vi "GUI_kHz_AlpaoWFS_broken.vi"() -> ()   [LabVIEW 2020]
uses:
  Shared/GUI_Template/GUI_master/tcp new data cluster.ctl
  <vilib>/vision/NI_Vision_Development_Module.lvlib
  <vilib>/vision/Image Controls.llb/IMAQ Image.ctl
  Shared/GUI_Template/GUI_master/tcp_new_data_event.ctl
panel:
  out "SpatialImage::1":T1(plugin-control) caption="Spatial Image"
  out "retrievedFrogTrace::1":T1(plugin-control) caption="Retrieved Frog Trace"
  out "frogTrace::1":T1(plugin-control) caption="FROG Trace"
  in  "cameraselect::1":enum16{"temporal CAM", "spatial CAM"}(ring) caption="Select Camera"
  in  "exposure::1":dbl=0.001 caption="Exposure" min=0.001 max=10000.0 format="%_4p"
  in  "triggermode::1":bool caption="Blank Button"
  in  "Select device":string(combo)="kHz_WFS_Alpao"
  out "tcp data event 2":T2
  out "Tank":dbl(slide) scale=0.0..255.0 scale format="%#_6p"
  out "Rotated_spatial":T1(plugin-control) caption="Raw image"
  out "error out":errorcluster
  in  "UDP error message":string
  in  "Refresh Button":bool
  out "GUIdevice 1":string="kHz_WFS_Alpao"
  in  "insert tag":bool=TRUE
  in  "stop":bool
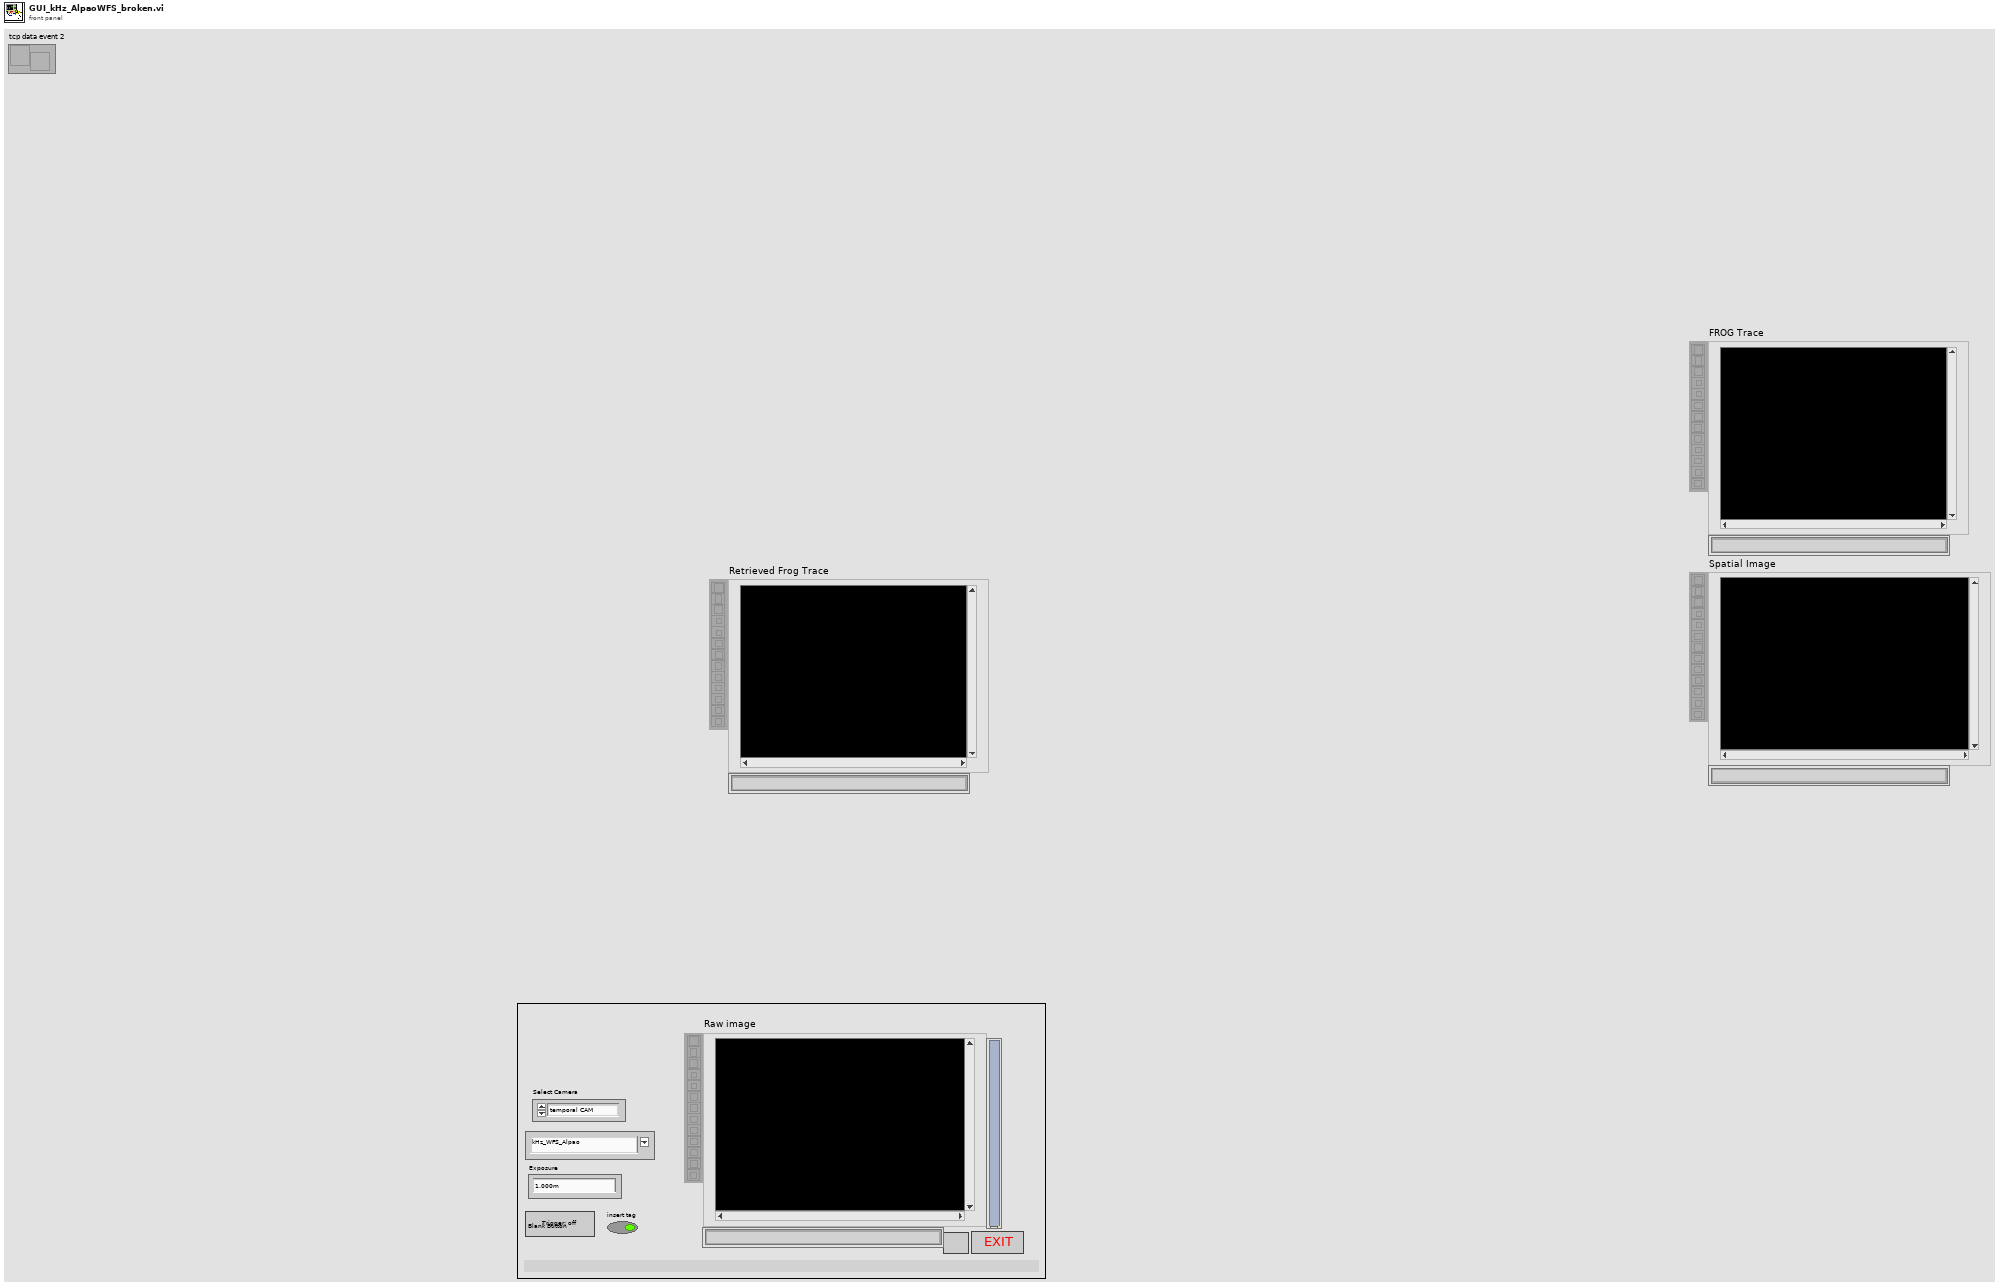
[diagram p1: front panel]
types:
  T1 = typedef "IMAQ Image.ctl" = refnum<image>
  T2 = typedef "tcp_new_data_event.ctl" = refnum<user-event>
  T3 = enum32{"invalid app kind", "Development System", "Run Time System", "Student Edition", "Embedded LabVIEW", "Evaluation", "Custom"}
  T4 = typedef "tcp new data cluster.ctl" = cluster{"EventEnum":enum16{"new data", "connection status update"}, "Device name":string}
  T5 = enum32{"Invalid", "Standard", "Closed", "Hidden", "Minimized", "Maximized"}
  T6 = cluster{"Left":i32, "Top":i32, "Right":i32, "Bottom":i32}
  T7 = cluster{"Core":cluster{"Current VI Reference":refnum<vi>, "Close Panel on Exit?":bool}, "Your Boolean data":bool, "Your string data":string, "SuperGUI":cluster{"STOP queue":refnum<queue>, "SuperGUI ref":refnum<vi>, "event reg":refnum<event-registration>}, "Images":cluster{"frogTrace::1":T1, "retrievedFrogTrace::1":T1, "SpatialImage::1":T1, "rotated_Temporal":T1, "rotated_Spatial":T1}}
  T8 = cluster{"frogTrace::1":T1, "retrievedFrogTrace::1":T1, "SpatialImage::1":T1, "rotated_Temporal":T1, "rotated_Spatial":T1}
  T9 = cluster{"STOP queue":refnum<queue>, "SuperGUI ref":refnum<vi>, "event reg":refnum<event-registration>}
  T10 = cluster{"Current VI Reference":refnum<vi>, "Close Panel on Exit?":bool}
  T11 = typedef "Image Type" = u32
  T12 = cluster{"histogram":u32[], "Minimal Value":sgl, "Maximal Value":sgl, "Starting Value":sgl, "Interval Width":sgl, "Mean Value":sgl, "Standard  Variation":sgl, "Area (pixels)":i32}
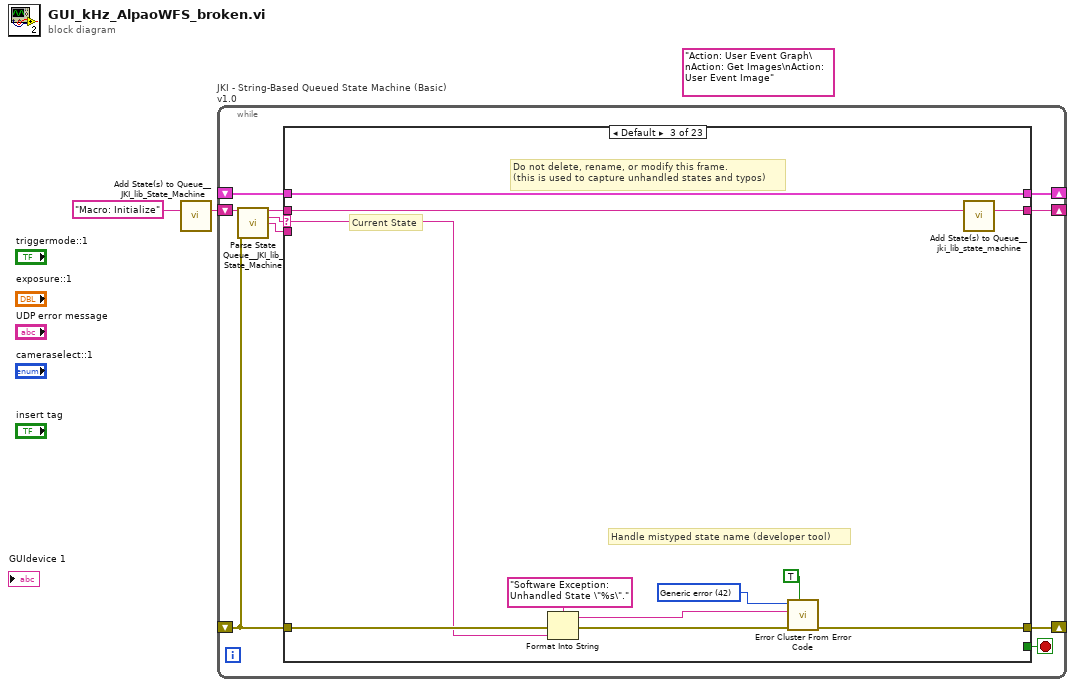
[diagram p0: block diagram]
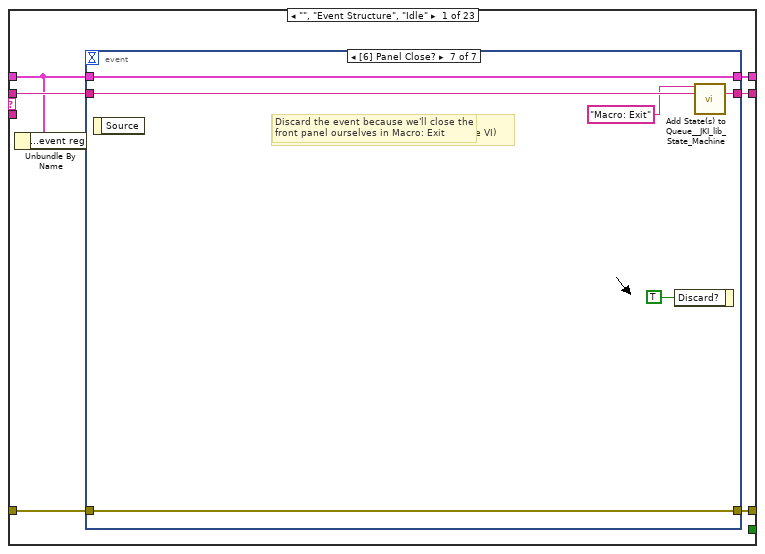
[diagram p2: hidden frame]
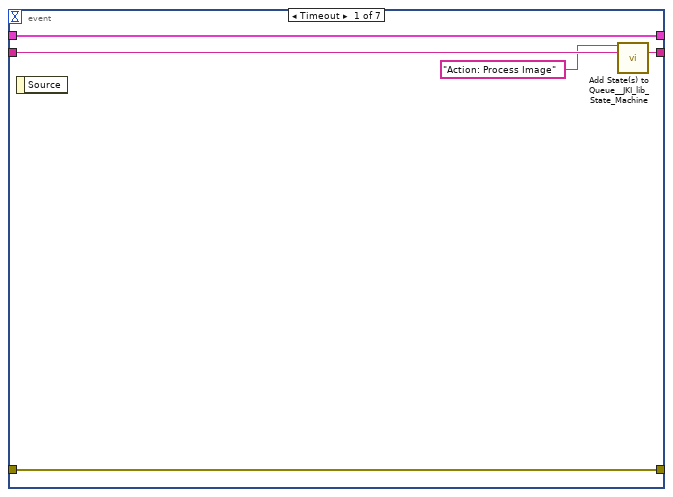
[diagram p3: hidden frame]
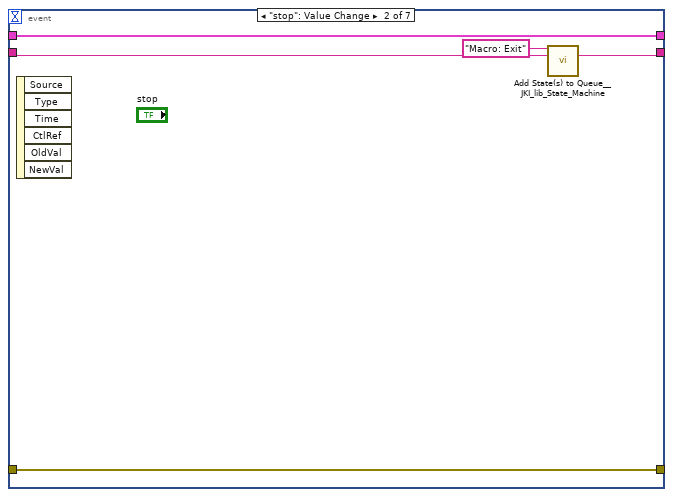
[diagram p4: hidden frame]
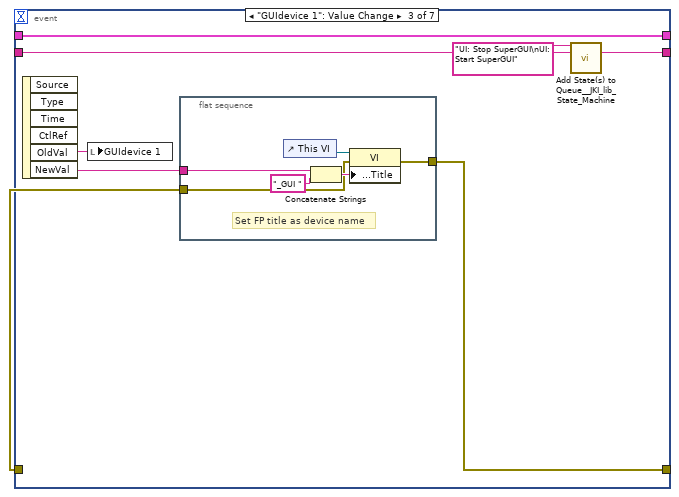
[diagram p5: hidden frame]
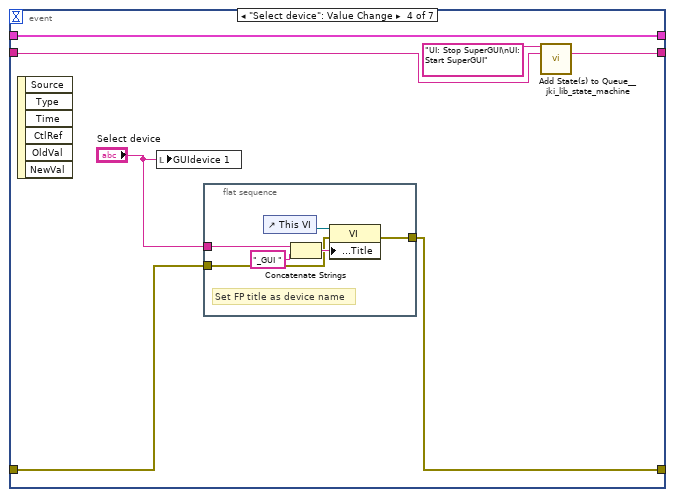
[diagram p6: hidden frame]
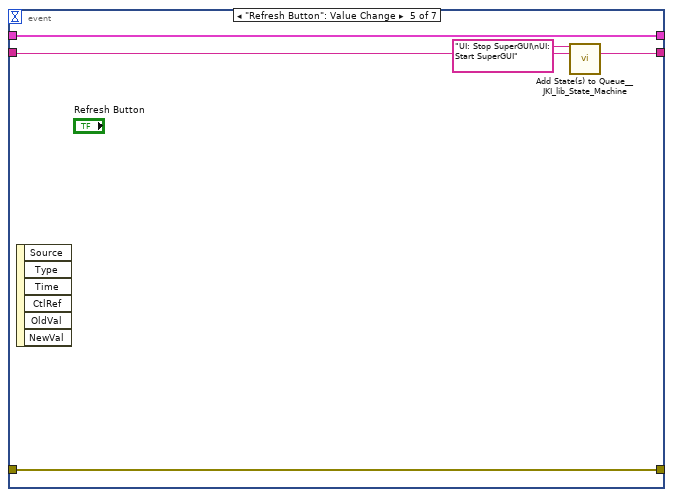
[diagram p7: hidden frame]
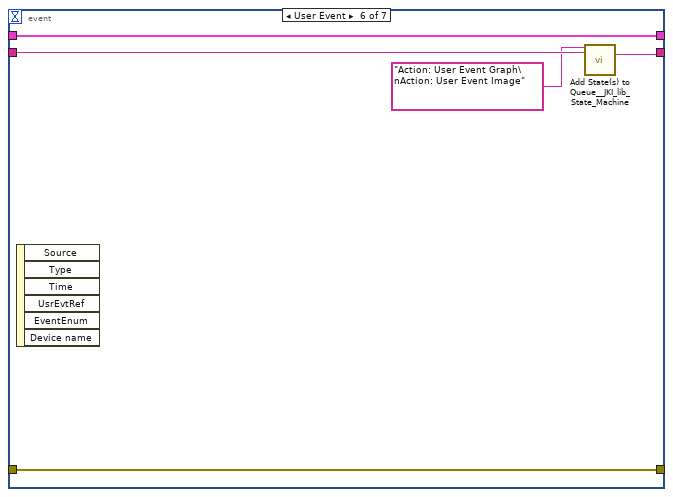
[diagram p8: hidden frame]
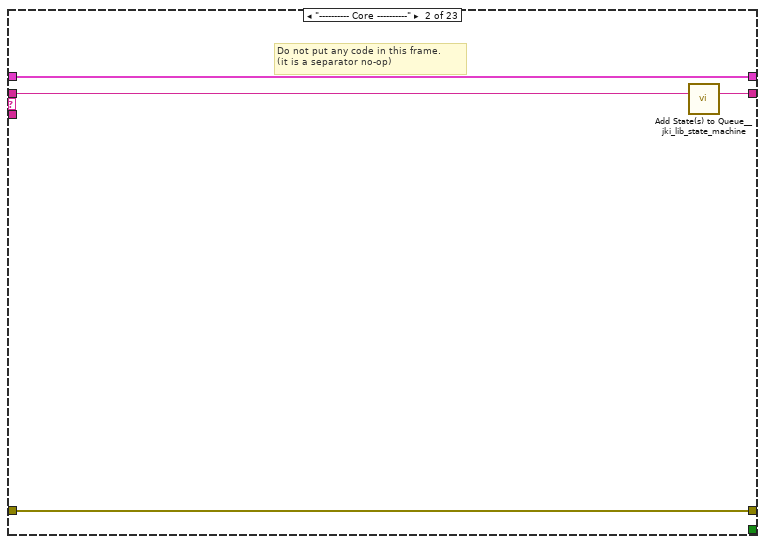
[diagram p9: hidden frame]
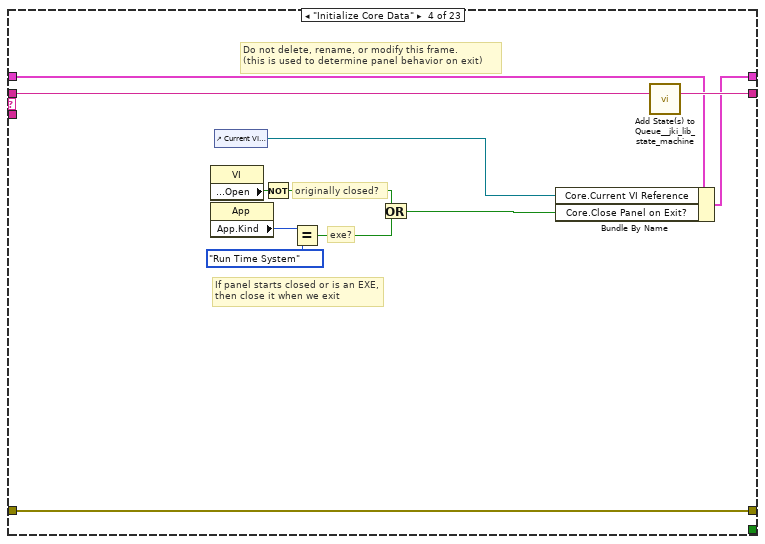
[diagram p10: hidden frame]
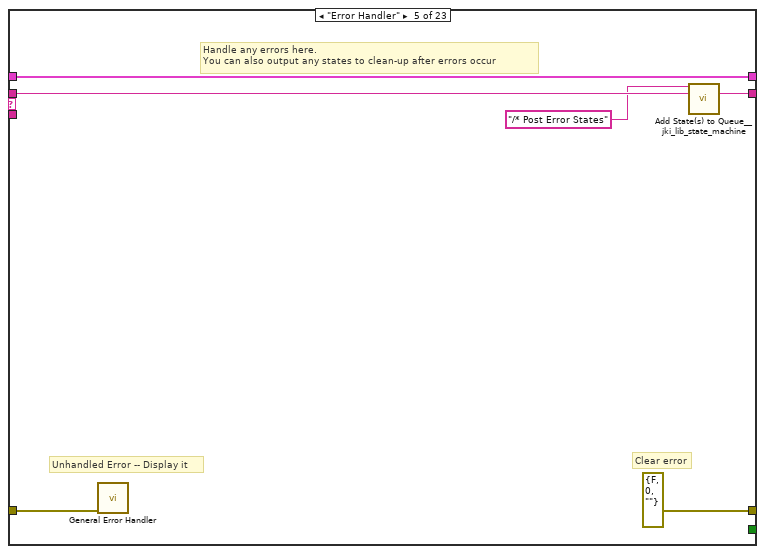
[diagram p11: hidden frame]
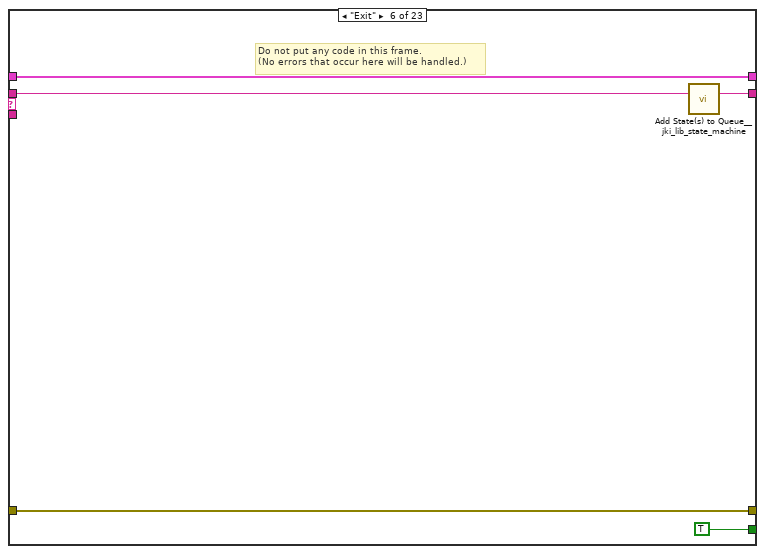
[diagram p12: hidden frame]
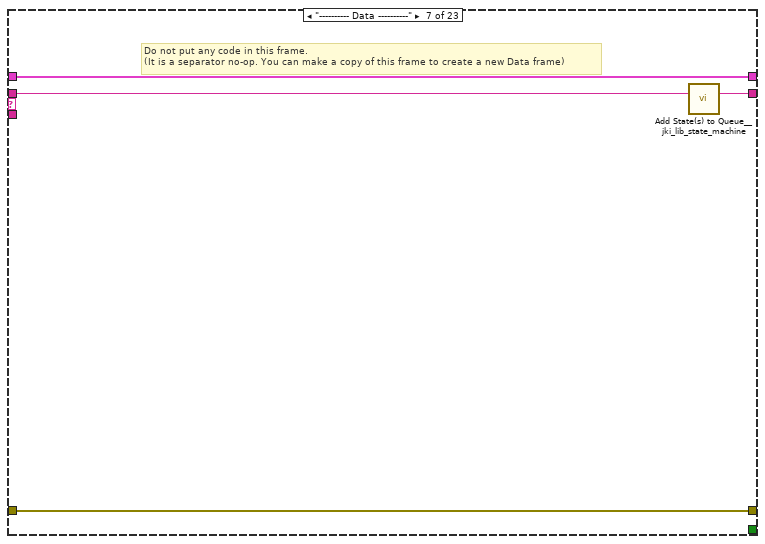
[diagram p13: hidden frame]
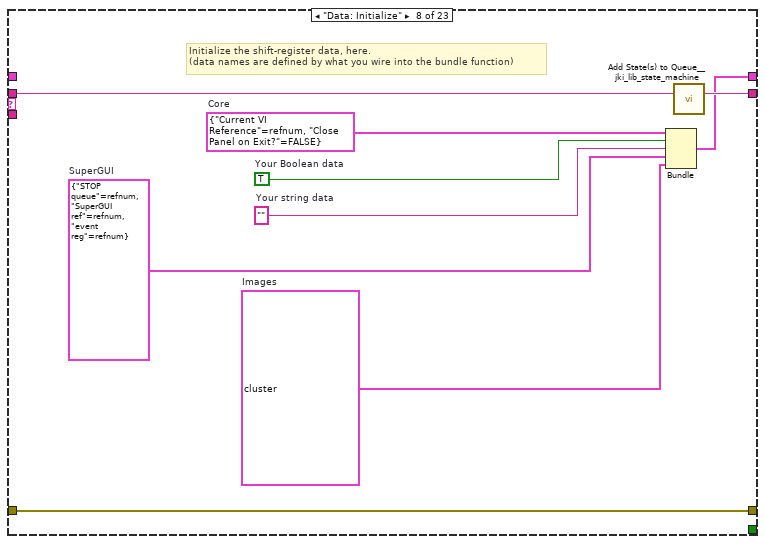
[diagram p14: hidden frame]
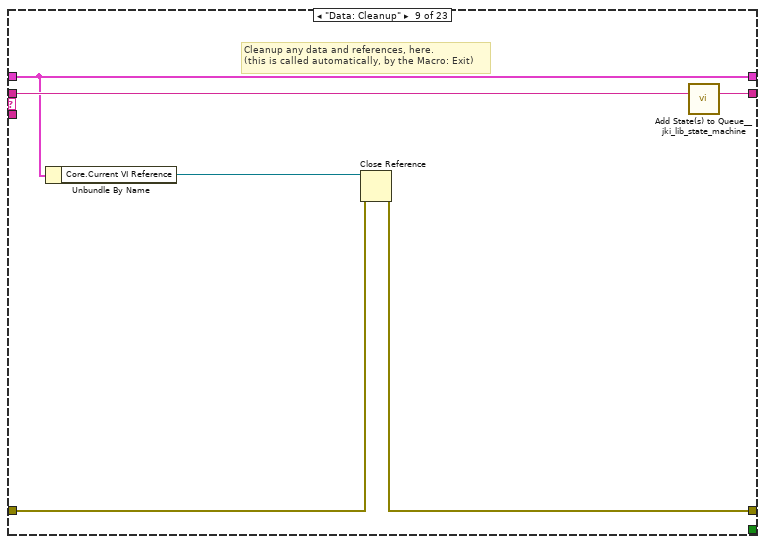
[diagram p15: hidden frame]
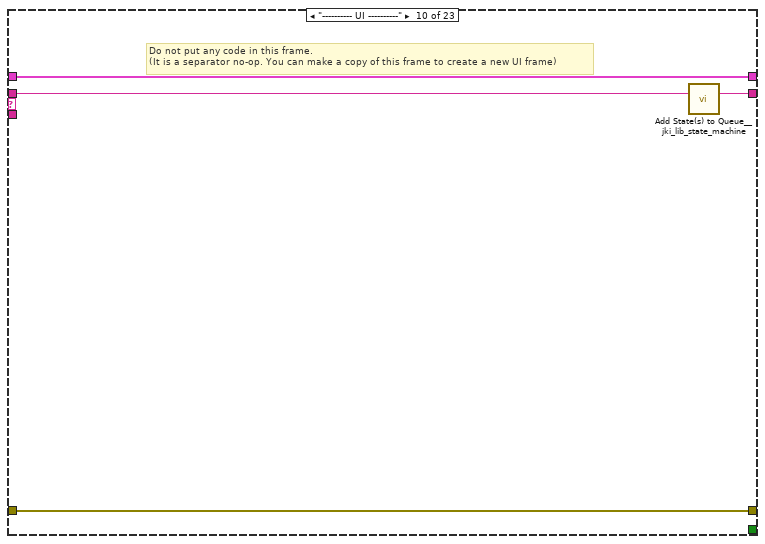
[diagram p16: hidden frame]
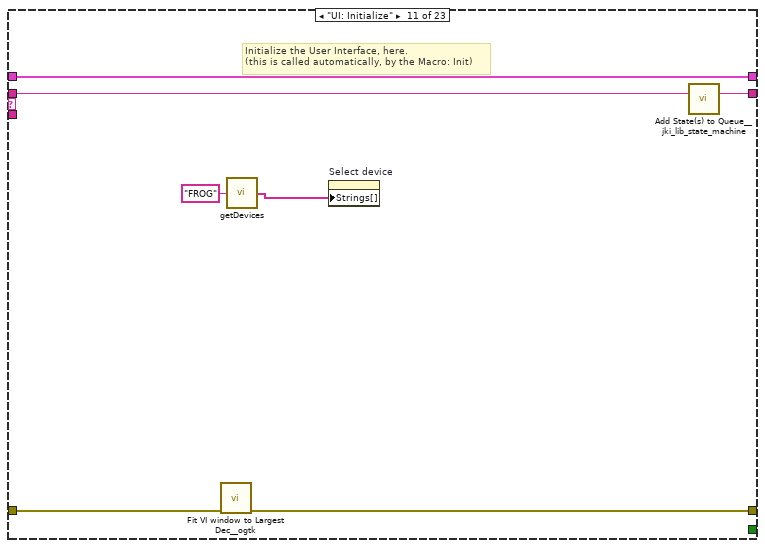
[diagram p17: hidden frame]
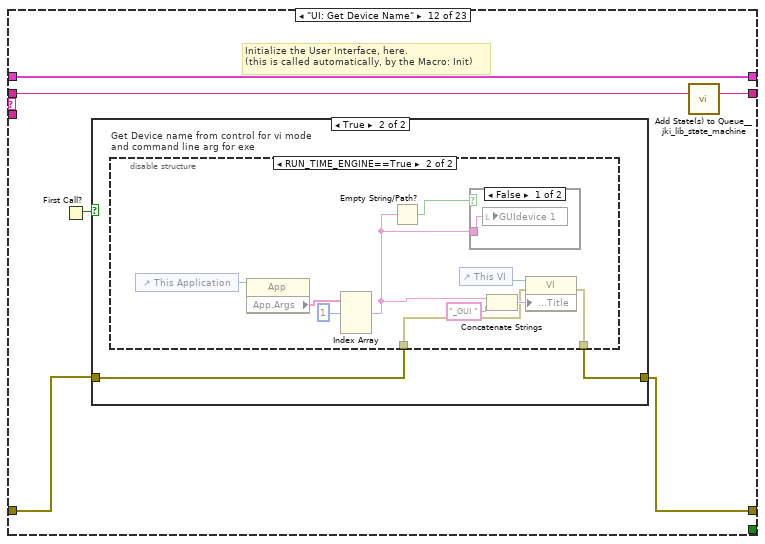
[diagram p18: hidden frame]
diagram:
  (unwired) "Action: User Event Graph\nAction: Get Images\nAction: User Event Image" ("State(s) in Front (\"\")")
  n1 = call <vilib>:"Add State(s) to Queue__JKI_lib_State_Machine.vi"("State(s) in (\"\")"="Macro: Initialize") -> ("States Out"=w2:string)  [unwired: 14 in]
  n2 = while "JKI - String-Based Queued State Machine (Basic) v1.0" {
    shift-right: [w5] -> _
    shift-left: _ -> [w4]
    shift-right: [w8] -> _
    shift-left: _ -> [w3]
    shift-right: [w7] -> _
    shift-left: w2 -> [w9]
    stop <- w6 stop-if-true
    n3 = call <vilib>:"Parse State Queue__JKI_lib_State_Machine.vi"("State Queue"=w9, "Error In (no error)"=w3) -> ("Remaining States"=w11:string, "Current State"=w12:string, "Arguments"=w10:string)  [unwired: 11 in]
    n4 = case shown="Default" w12 {
      selector: w12 -> [_ _ w75 _ _ _ _ _ _ _ _ _ _ _ _ _ _ _ _ _ _ _ _]
      tunnel: w11 -> [w18 w74 w79 w97 w103 w108 w112 w121 w127 w131 w138 w144 w181 w189 w195 w206 w230 w235 w245 w249 w253 w273 w288]
      tunnel: w10 -> [_ _ _ _ _ _ _ _ _ _ _ _ _ _ w190 w201 _ _ _ _ _ _ _]
      tunnel: w4 -> [w13 w71 w77 w87 w100 w106 w109 _ w123 w128 w136 w142 w161 w184 w193 w200 w227 w232 w237 w246 w250 w255 w276]
      tunnel: [w16 w72 w81 w95 errorcluster {"status"=FALSE, "code"=0, "source"=""} ("error out") w105 w110 w119 w124 w129 w134 w139 w168 w185 w191 w203 w228 w233 w243 w247 w251 w271 w286] -> w8
      tunnel: w3 -> [w15 w72 w80 w95 w99 w105 w110 w119 w125 w129 w135 w140 w169 w186 w192 w204 w228 w233 w243 w247 w251 w271 w286]
      tunnel: [w17 w73 w78 w96 w102 w107 w111 w120 w126 w130 w137 w143 w180 w188 w194 w205 w229 w234 w244 w248 w252 w272 w287] -> w7
      tunnel: [_ _ _ _ _ TRUE _ _ _ _ _ _ _ _ _ _ _ _ _ _ _ _ _] -> w6
      tunnel: [w14 w71 w77 w86 w100 w106 w109 w113 w123 w128 w136 w142 w160 w184 w193 w200 w227 w232 w237 w246 w250 w254 w276] -> w5
      frame "", "Event Structure", "Idle" {
        n5 = Unbundle By Name(w13) -> ()  [unwired: 1 out]
        n6 = event shown="[6] Panel Close?" {
          selector: _ -> [_ _ _ _ _ _ _]
          dyn-events: _ -> [_ _ _ _ _ _ _]
          timeout: _ -> [_ _ _ _ _ _ _]
          tunnel: w18 -> [w23 w26 w32 w44 w57 w63 w70]
          tunnel: [w22 w25 w31 w43 w56 w62 w69] -> w17
          tunnel: w13 -> [w20 w28 w35 w48 w59 w64 w67]
          tunnel: [w21 w27 w33 w46 w58 w60 w68] -> w16
          tunnel: w15 -> [w21 w27 w34 w47 w58 w60 w68]
          tunnel: [w20 w28 w35 w48 w59 w64 w67] -> w14
          event Timeout {
            n7 = event-data() -> ()  [unwired: 1 in, 1 out]
            n8 = call <vilib>:"Add State(s) to Queue__JKI_lib_State_Machine.vi"("State(s) in Front (\"\")"="Action: Process Image" ("State(s) in Front (\"\")"), "State(s) in (\"\")"=w23) -> ("States Out"=w22:string)  [unwired: 13 in]
          }
          event "stop": Value Change {
            n9 = event-data() -> ()  [unwired: 1 in, 6 out]
            n10 = call <vilib>:"Add State(s) to Queue__JKI_lib_State_Machine.vi"("State(s) in Front (\"\")"="Macro: Exit", "State(s) in (\"\")"=w26) -> ("States Out"=w25:string)  [unwired: 13 in]
          }
          event "GUIdevice 1": Value Change {
            n11 = event-data() -> ("NewVal"=w29:string)  [unwired: 1 in, 5 out]
            n12 = local write "GUIdevice 1"(w29) -> ()
            n13 = flat-sequence {
              tunnel: [w38] -> w33
              tunnel: w34 -> [w37]
              tunnel: w29 -> [w36]
              frame #0 {
                # "Set FP title as device name"
                n14 = control-ref of="This VI"() -> (w41:refnum<vi>)
                n15 = Concatenate Strings(w36, "_GUI ") -> (w40:string)
                n16 = property class="VI"(reference=w41, error in=w37, "Front Panel.Title"=w40) -> (error out=w38:errorcluster)  [unwired: 1 out]
              }
            }
            n17 = call <vilib>:"Add State(s) to Queue__JKI_lib_State_Machine.vi"("State(s) in Front (\"\")"="UI: Stop SuperGUI\nUI: Start SuperGUI", "State(s) in (\"\")"=w32) -> ("States Out"=w31:string)  [unwired: 13 in]
          }
          event "Select device": Value Change {
            n18 = event-data() -> ()  [unwired: 1 in, 6 out]
            n19 = local write "GUIdevice 1"("Select device") -> ()
            n20 = flat-sequence {
              tunnel: [w51] -> w46
              tunnel: w47 -> [w50]
              tunnel: "Select device" -> [w49]
              frame #0 {
                # "Set FP title as device name"
                n21 = control-ref of="This VI"() -> (w54:refnum<vi>)
                n22 = Concatenate Strings(w49, "_GUI ") -> (w53:string)
                n23 = property class="VI"(reference=w54, error in=w50, "Front Panel.Title"=w53) -> (error out=w51:errorcluster)  [unwired: 1 out]
              }
            }
            n24 = call <vilib>:"Add State(s) to Queue__jki_lib_state_machine.vi"("State(s) in Front (\"\")"="UI: Stop SuperGUI\nUI: Start SuperGUI", "State(s) in (\"\")"=w44) -> ("States Out"=w43:string)  [unwired: 13 in]
          }
          event "Refresh Button": Value Change {
            n25 = event-data() -> ()  [unwired: 1 in, 6 out]
            n26 = call <vilib>:"Add State(s) to Queue__JKI_lib_State_Machine.vi"("State(s) in Front (\"\")"="UI: Stop SuperGUI\nUI: Start SuperGUI", "State(s) in (\"\")"=w57) -> ("States Out"=w56:string)  [unwired: 13 in]
          }
          event User Event {
            n27 = event-data() -> ()  [unwired: 1 in, 6 out]
            n28 = call <vilib>:"Add State(s) to Queue__JKI_lib_State_Machine.vi"("State(s) in Front (\"\")"="Action: User Event Graph\nAction: User Event Image" ("State(s) in Front (\"\")"), "State(s) in (\"\")"=w63) -> ("States Out"=w62:string)  [unwired: 13 in]
          }
          event Panel Close? {
            # "Discard the event because we'll close the front panel ourselves in Macro: Exit"
            # "Close Panel button (pressed) Event\n(this executes Macro: Exit to terminate the VI)"
            n29 = event-data() -> ()  [unwired: 1 in, 1 out]
            n30 = event-data("Discard?"=TRUE) -> ()  [unwired: 1 in, 1 out]
            n31 = call <vilib>:"Add State(s) to Queue__JKI_lib_State_Machine.vi"("State(s) in Front (\"\")"="Macro: Exit", "State(s) in (\"\")"=w70) -> ("States Out"=w69:string)  [unwired: 13 in]
          }
        }
      }
      frame "---------- Core ----------" {
        # "Do not put any code in this frame.\n(it is a separator no-op)"
        n32 = call <vilib>:"Add State(s) to Queue__jki_lib_state_machine.vi"("State(s) in (\"\")"=w74) -> ("States Out"=w73:string)  [unwired: 14 in]
      }
      frame Default {
        w84 = 42 items=["No error", "Argument error", "Memory is full", "Out of zone", "End of file", "File already open", "Generic file I/O error", "File not found", "File permission error", "Disk is full", "Duplicate path", "Too many files open", "System feature not enabled", "Resource file not found", "Cannot add resource", "Resource not found", "Image not found", "Image memory error", "Pen does not exist", "Config type invalid", "Config token not found", "Config parse error", "Config memory error", "Bad external code format", "Bad external code offset", "External code not present", "Null window", "Destroy window error", "Null menu", "Print aborted", "Bad print record", "Print driver error", "Windows error during printing", "Memory error during printing", "Print dialog error", "Generic print error", "Invalid device refnum", "Device not found", "Device parameter error", "Device unit error", "Cannot open device", "Device call aborted", "Generic error", "Cancelled by user", "Object ID too low", "Object ID too high", "Object not in heap", "Unknown heap", "Unknown object (invalid DefProc)", "Unknown object (DefProc not in table)", "Message out of range", "Invalid (null) method", "Unknown message", "Manager call not supported", "Bad address", "Network operation in progress", "Network operation timed out", "Connection is busy", "Network attribute not supported", "Network error", "Address in use", "System out of memory", "Connection aborted", "Connection refused", "Not connected", "Already connected", "Connection closed", "Initialization error (interapplication manager)", "Bad occurrence", "Wait on unbound occurrence handler", "Occurrence queue overflow", "Datalog type conflict", "Unused", "Unrecognized type (interapplication manager)", "Memory corrupt", "Failed to make temporary DLL", "Old CIN version", "Drag socket not found", "Failed to load drop-object", "Failed to register OLE object", "Failed to release OLE object", "Format specifier type mismatch", "Unknown format specifier", "Too few format specifiers", "Too many format specifiers", "Scan failed", "Newer CIN version", "Error converting to variant", "Runtime menu error", "Password tampered", "Variant attribute not found", "Incompatible variant data type", "Event data is not available", "Event Store is not present", "Occurrence is not found", "Event Queue is not created", "Event info is not available", "Refnum passed is NULL", "Error retrieving Class GUID", "Error retrieving CoClass GUID", "Error retrieving TypeLib GUID.", "Bad built application magic bytes.", "Specific driver is different from the specific driver associated with the Logical Name.", "There is no session opened to the class driver.", "Max Error", "MAX - Error with config objects", "MAX - Error loading configuration", "MAX - Group not supported"]
        # "Current State"
        # "Do not delete, rename, or modify this frame.\n(this is used to capture unhandled states and typos)"
        # "Handle mistyped state name (developer tool)"
        n33 = Format Into String(format string="Software Exception: Unhandled State \"%s\"." ("message"), error in=w80, w75) -> (resulting string=w83:string, error out=w82:errorcluster)  [unwired: 1 in]
        n34 = call <vilib>:"Error Cluster From Error Code.vi"("show call chain? (False)"=TRUE, "error in (no error)"=w82, "error message (\"\")"=w83, "error code (0)"=w84) -> ("error out"=w81:errorcluster)  [unwired: 5 in]
        n35 = call <vilib>:"Add State(s) to Queue__jki_lib_state_machine.vi"("State(s) in (\"\")"=w79) -> ("States Out"=w78:string)  [unwired: 14 in]
      }
      frame "Initialize Core Data" {
        # "Do not delete, rename, or modify this frame.\n(this is used to determine panel behavior on exit)"
        # "originally closed?"
        # "exe?"
        # "If panel starts closed or is an EXE, then close it when we exit"
        n36 = property class="VI"() -> ("Front Panel.Open"=w94:bool)  [unwired: 2 in, 2 out]
        n37 = property class="App"() -> ("App.Kind"=w93:T3)  [unwired: 2 in, 2 out]
        n38 = control-ref of="Current VI Reference"() -> (w88:refnum<vi>)
        n39 = Not(x=w94) -> (.not. x?=w91:bool)
        n40 = Equal?(x=w93, y=T3."Run Time System" ("Application:Kind")) -> (x = y?=w90:bool)
        n41 = Or(x=w91, y=w90) -> (x .or. y?=w89:bool)
        n42 = Bundle By Name(cluster=w87, "Core.Current VI Reference"=w88, "Core.Close Panel on Exit?"=w89) -> (w86:T7)
        n43 = call <vilib>:"Add State(s) to Queue__jki_lib_state_machine.vi"("State(s) in (\"\")"=w97) -> ("States Out"=w96:string)  [unwired: 14 in]
      }
      frame "Error Handler" {
        # "Unhandled Error -- Display it"
        # "Handle any errors here.\nYou can also output any states to clean-up after errors occur"
        # "Clear error"
        n44 = call <vilib>:"General Error Handler.vi"("error in (no error)"=w99) -> ()  [unwired: 10 in, 5 out]
        n45 = call <vilib>:"Add State(s) to Queue__jki_lib_state_machine.vi"("State(s) in Front (\"\")"="/* Post Error States", "State(s) in (\"\")"=w103) -> ("States Out"=w102:string)  [unwired: 13 in]
      }
      frame "Exit" {
        # "Do not put any code in this frame.\n(No errors that occur here will be handled.)"
        n46 = call <vilib>:"Add State(s) to Queue__jki_lib_state_machine.vi"("State(s) in (\"\")"=w108) -> ("States Out"=w107:string)  [unwired: 14 in]
      }
      frame "---------- Data ----------" {
        # "Do not put any code in this frame.\n(It is a separator no-op. You can make a copy of this frame to create a new Data frame)"
        n47 = call <vilib>:"Add State(s) to Queue__jki_lib_state_machine.vi"("State(s) in (\"\")"=w112) -> ("States Out"=w111:string)  [unwired: 14 in]
      }
      frame "Data: Initialize" {
        w114 = T8 {"frogTrace::1"="remote image 000000001B06411C", "retrievedFrogTrace::1"="remote image 000000001B06411C", "SpatialImage::1"="remote image 000000001B06411C", "rotated_Temporal"=refnum, "rotated_Spatial"=refnum}  # Images
        w115 = T9 {"STOP queue"=refnum, "SuperGUI ref"=refnum, "event reg"=refnum}  # SuperGUI
        w116 = T10 {"Current VI Reference"=refnum, "Close Panel on Exit?"=FALSE}  # Core
        w118 = TRUE  # Your Boolean data
        w117 = ""  # Your string data
        # "Initialize the shift-register data, here.\n(data names are defined by what you wire into the bundle function)"
        n48 = Bundle("Core"=w116, "Your Boolean data"=w118, "Your string data"=w117, "SuperGUI"=w115, "Images"=w114) -> (w113:T7)  [unwired: 1 in]
        n49 = call <vilib>:"Add State(s) to Queue__jki_lib_state_machine.vi"("State(s) in (\"\")"=w121) -> ("States Out"=w120:string)  [unwired: 14 in]
      }
      frame "Data: Cleanup" {
        # "Cleanup any data and references, here.\n(this is called automatically, by the Macro: Exit)"
        n50 = Unbundle By Name(w123) -> ("Core.Current VI Reference"=w122:refnum<vi>)
        n51 = Close Reference(reference=w122, error in (no error)=w125) -> (error out=w124:errorcluster)
        n52 = call <vilib>:"Add State(s) to Queue__jki_lib_state_machine.vi"("State(s) in (\"\")"=w127) -> ("States Out"=w126:string)  [unwired: 14 in]
      }
      frame "---------- UI ----------" {
        # "Do not put any code in this frame.\n(It is a separator no-op. You can make a copy of this frame to create a new UI frame)"
        n53 = call <vilib>:"Add State(s) to Queue__jki_lib_state_machine.vi"("State(s) in (\"\")"=w131) -> ("States Out"=w130:string)  [unwired: 14 in]
      }
      frame "UI: Initialize" {
        # "Initialize the User Interface, here.\n(this is called automatically, by the Macro: Init)"
        n54 = call <userlib>:"Fit VI window to Largest Dec__ogtk.vi"("error in (no error)"=w135) -> ("error out"=w134:errorcluster)  [unwired: 5 in, 1 out]
        n55 = call "getDevices.vi"("Device Class"="FROG") -> ("All Devices"=w132:string[])
        n56 = property on="Select device" class="CmbBox"("Strings[]"=w132) -> ()  [unwired: 2 in, 2 out]
        n57 = call <vilib>:"Add State(s) to Queue__jki_lib_state_machine.vi"("State(s) in (\"\")"=w138) -> ("States Out"=w137:string)  [unwired: 14 in]
      }
      frame "UI: Get Device Name" {
        # "Initialize the User Interface, here.\n(this is called automatically, by the Macro: Init)"
        n58 = First Call?() -> (First Call?: T/F=w141:bool)
        n59 = case shown="True" w141 {
          tunnel: w140 -> [w145 w147]
          tunnel: [w145 w146] -> w139
          frame False {
          }
          frame True {
            n60 = disable-structure "Get Device name from control for vi mode\nand command line arg for exe" shown="RUN_TIME_ENGINE==True" {
              disable-tunnel: w147 -> [w148 w150]
              disable-tunnel: [w148 w149] -> w146
              frame condition #0 (active) {
              }
              frame condition #1 {
                n61 = control-ref of="This Application"() -> (w158:refnum<vi>)
                n62 = property class="App"(reference=w158) -> ("App.Args"=w157:string[])  [unwired: 1 in, 2 out]
                n63 = Index Array(array=w157, index #1=1 ("index")) -> (element #1=w151:string)  [unwired: 2 in, 2 out]
                n64 = Empty String/Path?(string/path=w151) -> (empty?=w155:bool)
                n65 = control-ref of="This VI"() -> (w154:refnum<vi>)
                n66 = case shown="False" w155 {
                  tunnel: w151 -> [w159 _]
                  frame False {
                    n67 = local write "GUIdevice 1"(w159) -> ()
                  }
                  frame True {
                  }
                }
                n68 = Concatenate Strings(w151, "_GUI ") -> (w153:string)
                n69 = property class="VI"(reference=w154, error in=w150, "Front Panel.Title"=w153) -> (error out=w149:errorcluster)  [unwired: 1 out]
              }
            }
          }
        }
        n70 = call <vilib>:"Add State(s) to Queue__jki_lib_state_machine.vi"("State(s) in (\"\")"=w144) -> ("States Out"=w143:string)  [unwired: 14 in]
      }
      frame "UI: Start SuperGUI" {
        # "create stop queue for supergui and its clones"
        # "x100 abort will be dependent on caller VI\nx80 abort will be independent of caller vi, this will abort vi when labview is closed."
        # "Start SuperGUI asynchronous way"
        n71 = vi-ref "GUI_Master_subvi_reentrant_queues.vi"() -> (w167:refnum<vi>)
        n72 = property class="VI"(reference=w167) -> ("Path"=w166:path)  [unwired: 1 in, 2 out]
        n73 = Create User Event(user event datatype=T4 {"EventEnum"=enum."new data", "Device name"="Device name"} ("New Event"), error in=w169) -> (user event=w164:refnum<user-event>, error out=w173:errorcluster)
        "tcp data event 2" <- w164
        n74 = control-ref of="This Application"() -> (w172:refnum<vi>)
        n75 = control-ref of="This VI"() -> (w171:refnum<vi>)
        n76 = Open VI Reference(type specifier VI Refnum (for type only)=refnum<vi> refnum, vi path=w166, options=256) -> (vi reference=w179:refnum<vi>, error out=w178:errorcluster)  [unwired: 3 in]
        n77 = register-events(w164) -> (reference out=w163:refnum<event-registration>)  [unwired: 2 in, 1 out]
        n78 = call "supergui create stop queue.vi"() -> ("STOP Queue out"=w175:refnum<queue>)  [unwired: 11 in]
        n79 = Current VI's Menubar() -> (w170:refnum<k9>)
        n80 = call-by-ref "Start Asynchronous Call"(reference=w179, error in=w178, "STOP Queue in"=w175, "This Application"=w172, 8:"error in (no error)"=w173, "tcp data event"=w164, "Caller menu reference"=w170, "Caller VI ref"=w171) -> (reference out=w165:refnum<vi>, error out=w168:errorcluster)  [unwired: 5 in, 1 out]
        n81 = Bundle By Name(cluster=w161, "SuperGUI.event reg"=w163, "SuperGUI.SuperGUI ref"=w165, "SuperGUI.STOP queue"=w175) -> (w160:T7)
        n82 = call <vilib>:"Add State(s) to Queue__jki_lib_state_machine.vi"("State(s) in Front (\"\")"="Action: Get Images" ("State(s) in Front (\"\")"), "State(s) in (\"\")"=w181) -> ("States Out"=w180:string)  [unwired: 13 in]
      }
      frame "UI: Stop SuperGUI" {
        # "Stop Supergui Clone and wait until it exit properly"
        n83 = Unbundle By Name(w184) -> ("SuperGUI.SuperGUI ref"=w182:refnum<vi>, "SuperGUI.STOP queue"=w183:refnum<queue>)
        n84 = Release Queue(queue=w183, error in (no error)=w186) -> (error out=w187:errorcluster)  [unwired: 1 in, 2 out]
        n85 = call-by-ref "Wait On Asynchronous Call"(reference=w182, error in=w187) -> ("error out"=w185:errorcluster)  [unwired: 11 in, 2 out]
        n86 = call <vilib>:"Add State(s) to Queue__jki_lib_state_machine.vi"("State(s) in (\"\")"=w189) -> ("States Out"=w188:string)  [unwired: 14 in]
      }
      frame "UI: Cursor Set" {
        # "Argument"
        # "Set and Unset Cursor Busy.\n(Usage: \"UI: Cursor Set >> Busy|Idle\")"
        n87 = case shown="\"Idle\", Default" w190 {
          tunnel: w192 -> [w197 w199]
          tunnel: [w196 w198] -> w191
          frame "Idle", Default {
            n88 = call <vilib>:"Unset Busy.vi"("error in (no error)"=w197) -> ("error out"=w196:errorcluster)  [unwired: 10 in]
          }
          frame "Busy" {
            n89 = call <vilib>:"Set Busy.vi"("error in (no error)"=w199) -> ("error out"=w198:errorcluster)  [unwired: 9 in, 1 out]
          }
        }
        n90 = call <vilib>:"Add State(s) to Queue__jki_lib_state_machine.vi"("State(s) in (\"\")"=w195) -> ("States Out"=w194:string)  [unwired: 14 in]
      }
      frame "UI: Front Panel State" {
        # "Argument"
        # "Set Front Panel Open or Closed\n(Usage: \"UI: Front Panel State >> Open|Close\")"
        n91 = Unbundle By Name(w200) -> ("Core.Current VI Reference"=w202:refnum<vi>)
        n92 = case shown="\"Open\", Default" w201 {
          tunnel: w204 -> [w210 w221]
          tunnel: [w211 w222] -> w203
          tunnel: w202 -> [_ _]
          frame "Open", Default {
            n93 = property class="VI"(error in=w210) -> (reference out=w208:refnum<vi>, error out=w209:errorcluster, "Front Panel.Open"=w207:bool)  [unwired: 1 in]
            n94 = case shown="False" w207 {
              tunnel: [w214 w217] -> w211
              tunnel: w209 -> [w213 w217]
              tunnel: w208 -> [w212 _]
              frame False {
                n95 = invoke class="VI" method="FP.Open"(reference=w212, error in=w213, "Activate"=TRUE, "State"=T5."Standard") -> (error out=w214:errorcluster)  [unwired: 1 in, 4 out]
              }
              frame True {
              }
            }
          }
          frame "Close" {
            n96 = property class="VI"(error in=w221) -> (reference out=w219:refnum<vi>, error out=w220:errorcluster, "Front Panel.Open"=w218:bool)  [unwired: 1 in]
            n97 = case shown="True" w218 {
              tunnel: [w223 w226] -> w222
              tunnel: w220 -> [w223 w225]
              tunnel: w219 -> [_ w224]
              frame False {
              }
              frame True {
                n98 = invoke class="VI" method="FP.Close"(reference=w224, error in=w225) -> (error out=w226:errorcluster)  [unwired: 1 in, 2 out]
              }
            }
          }
        }
        n99 = call <vilib>:"Add State(s) to Queue__jki_lib_state_machine.vi"("State(s) in (\"\")"=w206) -> ("States Out"=w205:string)  [unwired: 14 in]
      }
      frame "---------- Macro ----------" {
        # "Do not put any code in this frame.\n(It is a separator no-op. You can make a copy of this frame to create a new Macro frame)"
        n100 = call <vilib>:"Add State(s) to Queue__jki_lib_state_machine.vi"("State(s) in (\"\")"=w230) -> ("States Out"=w229:string)  [unwired: 14 in]
      }
      frame "Macro: Initialize" {
        # "Initialization Macro\n(This is called once, when the VI starts)"
        n101 = call <vilib>:"Add State(s) to Queue__jki_lib_state_machine.vi"("State(s) in Front (\"\")"="Data: Initialize\nInitialize Core Data\nUI: Initialize\nUI: Get Device Name\nUI: Start SuperGUI\nUI: Front Panel State >> Open", "State(s) in (\"\")"=w235) -> ("States Out"=w234:string)  [unwired: 13 in]
      }
      frame "Macro: Exit" {
        # "Exit Macro\n(This is called once, when the VI exits)"
        n102 = Unbundle By Name(w237) -> ("Core.Close Panel on Exit?"=w236:bool)
        n103 = Select(t="UI: Front Panel State >> Close", s=w236, f="") -> (s? t:f=w240:string)
        n104 = call <vilib>:"Add State(s) to Queue__jki_lib_state_machine.vi"("State(s) in (\"\")"=w240, "State(s) at Back (\"\")"="Data: Cleanup\nExit") -> ("States Out"=w238:string)  [unwired: 13 in]
        n105 = call <vilib>:"Add State(s) to Queue__jki_lib_state_machine.vi"("State(s) in Front (\"\")"=w238, "State(s) in (\"\")"=w245) -> ("States Out"=w244:string)  [unwired: 13 in]
      }
      frame "---------- New Category ----------" {
        # "Template Separator\n(You can make a copy of, or modify, this frame)"
        n106 = call <vilib>:"Add State(s) to Queue__jki_lib_state_machine.vi"("State(s) in (\"\")"=w249) -> ("States Out"=w248:string)  [unwired: 14 in]
      }
      frame "Action: User Event Graph" {
        n107 = call <vilib>:"Add State(s) to Queue__jki_lib_state_machine.vi"("State(s) in (\"\")"=w253) -> ("States Out"=w252:string)  [unwired: 14 in]
      }
      frame "Action: Get Images" {
        w267 = T11 0 items=["Grayscale (U8)", "Grayscale (I16)", "Grayscale (SGL)", "Complex (CSG)", "RGB (U32)", "HSL (U32)", "RGB (U64)", "Grayscale (U16)"] ("Image Type")
        w270 = T11 0 items=["Grayscale (U8)", "Grayscale (I16)", "Grayscale (SGL)", "Complex (CSG)", "RGB (U32)", "HSL (U32)", "RGB (U64)", "Grayscale (U16)"] ("Image Type")
        w261 = T11 0 items=["Grayscale (U8)", "Grayscale (I16)", "Grayscale (SGL)", "Complex (CSG)", "RGB (U32)", "HSL (U32)", "RGB (U64)", "Grayscale (U16)"] ("Image Type")
        w264 = T11 0 items=["Grayscale (U8)", "Grayscale (I16)", "Grayscale (SGL)", "Complex (CSG)", "RGB (U32)", "HSL (U32)", "RGB (U64)", "Grayscale (U16)"] ("Image Type")
        w265 = T11 0 items=["Grayscale (U8)", "Grayscale (I16)", "Grayscale (SGL)", "Complex (CSG)", "RGB (U32)", "HSL (U32)", "RGB (U64)", "Grayscale (U16)"] ("Image Type")
        n108 = call "IMAQ Create"("Image Name"="retrievedFrogTrace::1", "Image Type"=w264) -> ("New Image"=w259:T1)  [unwired: 3 in, 1 out]
        "retrievedFrogTrace::1" <- w259
        n109 = call "IMAQ Create"("Image Name"="frogTrace::1", "Image Type"=w265) -> ("New Image"=w260:T1)  [unwired: 3 in, 1 out]
        "frogTrace::1" <- w260
        n110 = call "IMAQ Create"("Image Name"="SpatialImage::1", "Image Type"=w261) -> ("New Image"=w258:T1)  [unwired: 3 in, 1 out]
        "SpatialImage::1" <- w258
        n111 = call "IMAQ Create"("Image Name"="rotated_Spatial", "Image Type"=w267) -> ("New Image"=w256:T1)  [unwired: 3 in, 1 out]
        n112 = call "IMAQ Create"("Image Name"="rotated_Temporal", "Image Type"=w270) -> ("New Image"=w257:T1)  [unwired: 3 in, 1 out]
        n113 = Bundle By Name(cluster=w255, "Images.SpatialImage::1"=w260, "Images.rotated_Spatial"=w259, "Images.SpatialImage::1"=w258, "Images.rotated_Temporal"=w257, "Images.rotated_Spatial"=w256) -> (w254:T7)
        n114 = call <vilib>:"Add State(s) to Queue__jki_lib_state_machine.vi"("State(s) in (\"\")"=w273) -> ("States Out"=w272:string)  [unwired: 14 in]
      }
      frame "Action: User Event Image" {
        n115 = Unbundle By Name(w276) -> ("Images.SpatialImage::1"=w275:T1, "Images.rotated_Spatial"=w274:T1)  [unwired: 2 out]
        n116 = call "IMAQ Rotate"("Maintain Size"=FALSE, "Angle (degrees)"=sgl 90.0, "Image Dst"=w274, "Image Src"=w275) -> ("error out"=w278:errorcluster, "Image Dst Out"=w281:T1)  [unwired: 6 in]
        n117 = call "IMAQ Histogram"("Image"=w275) -> ("Histogram Report"=w284:T12)  [unwired: 9 in, 1 out]
        n118 = call <vilib>:"Clear Errors.vi"("error in (no error)"=w278) -> ("error out"=w282:errorcluster)  [unwired: 5 in, 1 out]
        n119 = disable-structure shown="Enabled" {
          disable-tunnel: [w293 w294] -> w283
          disable-tunnel: w282 -> [w292 w295]
          disable-tunnel: w281 -> [w291 w294]
          disable-tunnel: [w289 w295] -> w280
          frame Disabled {
            (unwired) 384.0 ("Target.Y")
            (unwired) 288.0 ("Target.X")
            (unwired) cluster{"xhair size":dbl, "xhair size 2":dbl} {"xhair size"=275.0, "xhair size 2"=275.0} ("size")
            (unwired) u32 16774656 ("Color")
            n120 = call "draw crosshair imaq.vi"("error in (no error)"=w292, "Bounding Rectangle"=T6 {"Left"=0, "Top"=0, "Right"=0, "Bottom"=0}, "image in"=w291) -> ("error out"=w289:errorcluster, "image out"=w293:T1)  [unwired: 7 in]
          }
          frame Enabled {
          }
        }
        "Rotated_spatial" <- w283
        "error out" <- w280
        n121 = Unbundle By Name(w284) -> ("Maximal Value"=→"Tank":sgl)
        n122 = call <vilib>:"Add State(s) to Queue__jki_lib_state_machine.vi"("State(s) in (\"\")"=w288) -> ("States Out"=w287:string)  [unwired: 14 in]
      }
    }
  }
